vi "Set Transfer Line Valve Interlock Configuration.vi"(8 "error in (no error)":errorcluster, 9 "Manual Mode (False)":bool, 10 "Open? (False)":bool, 11 "Preparation Line in":refnum<class "Preparation Line.lvclass">) -> (0 "error out":errorcluster, 1 "Interlock Chain":refnum<class "Interlock Chain.lvclass">, 2 "Open? (False)":bool, 3 "Preparation Line out":refnum<class "Preparation Line.lvclass">)   [LabVIEW 2015, in "cRIO-Carbondioxide.lvlib" / "CO2-Actor.lvlib" / "Preparation Line.lvclass"]
uses:
  Preparation Line.lvclass
  Interlocks/Interlock Chain/Interlock Chain.lvclass
  Interlocks/Interlock/Interlock.lvclass
  Interlocks/Controls/Add IL to -Enumerator.ctl
  Transfer Line/Transfer Line.lvclass
  Interlocks/Interlock Sample/Interlock Sample.lvclass
  subs/Sample/Sample.lvclass
  CO2 Actor Messages/Ping Msg/Ping Msg.lvclass/Ping Msg.ctl
  <vilib>/ActorFramework/Message Enqueuer/Message Enqueuer.lvclass/Message Enqueuer.ctl
  Transfer Line/Transfer Line.lvclass/Transfer Line.ctl
  Interlocks/Interlock Chain/Interlock Chain.lvclass/Interlock Chain.ctl
  <vilib>/ActorFramework/Message Enqueuer/Enqueue.vi
  <vilib>/ActorFramework/Message Priority Queue/Priority Enqueue.vi
  subs/Sample/Read Sample From Container.vi
  CO2 Actor Messages/Ping Msg/Ping Msg.lvclass
  <vilib>/ActorFramework/Actor/Actor.lvclass
  CO2 Actor/CO2 Actor.lvclass
  cRIO-CO2/cRIO-CO2.lvclass
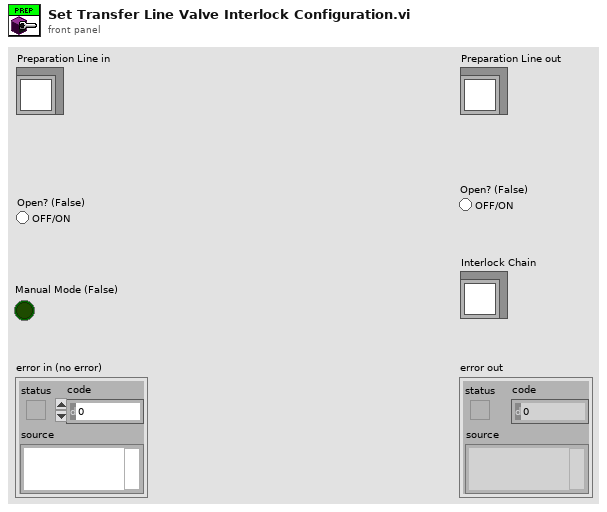
[diagram p1: front panel]
types:
  T1 = typedef "Add IL to -Enumerator.ctl" = enum16{"Deny", "Allow", "None"}
  T2 = typedef "Dedicated Enqueuers.ctl" = cluster{"Freezers":cluster{"Syringe":refnum<class "Message Enqueuer.lvclass">, "Tank 1":refnum<class "Message Enqueuer.lvclass">, "Tank 2":refnum<class "Message Enqueuer.lvclass">, "Tank 3":refnum<class "Message Enqueuer.lvclass">, "Tank 4":refnum<class "Message Enqueuer.lvclass">}, "Heaters":cluster{"Syringe":refnum<class "Message Enqueuer.lvclass">, "Piston":refnum<class "Message Enqueuer.lvclass">}, "Blowers":cluster{"Tank 1":refnum<class "Message Enqueuer.lvclass">, "Tank 2":refnum<class "Message Enqueuer.lvclass">, "Tank 3":refnum<class "Message Enqueuer.lvclass">, "Tank 4":refnum<class "Message Enqueuer.lvclass">, "Syringe":refnum<class "Message Enqueuer.lvclass">}, "Sample Line":refnum<class "Message Enqueuer.lvclass">, "Storage Line":refnum<class "Message Enqueuer.lvclass">, "Transfer Line":refnum<class "Message Enqueuer.lvclass">, "Syringe Stepper":refnum<class "Message Enqueuer.lvclass">, "Syringe Line":refnum<class "Message Enqueuer.lvclass">, "Capillary Line":refnum<class "Message Enqueuer.lvclass">, "Preparation Line":refnum<class "Message Enqueuer.lvclass">, "Turbo":refnum<class "Message Enqueuer.lvclass">, "Vacuum":refnum<class "Message Enqueuer.lvclass">, "He Line":refnum<class "Message Enqueuer.lvclass">, "Cylinder":refnum<class "Message Enqueuer.lvclass">}
  T3 = typedef "Sample Container.ctl" = cluster{"Sample In":refnum<k21>, "Sample Name":refnum<k21>, "Ti Cathode":refnum<k21>, "SampleQ":refnum<queue>}
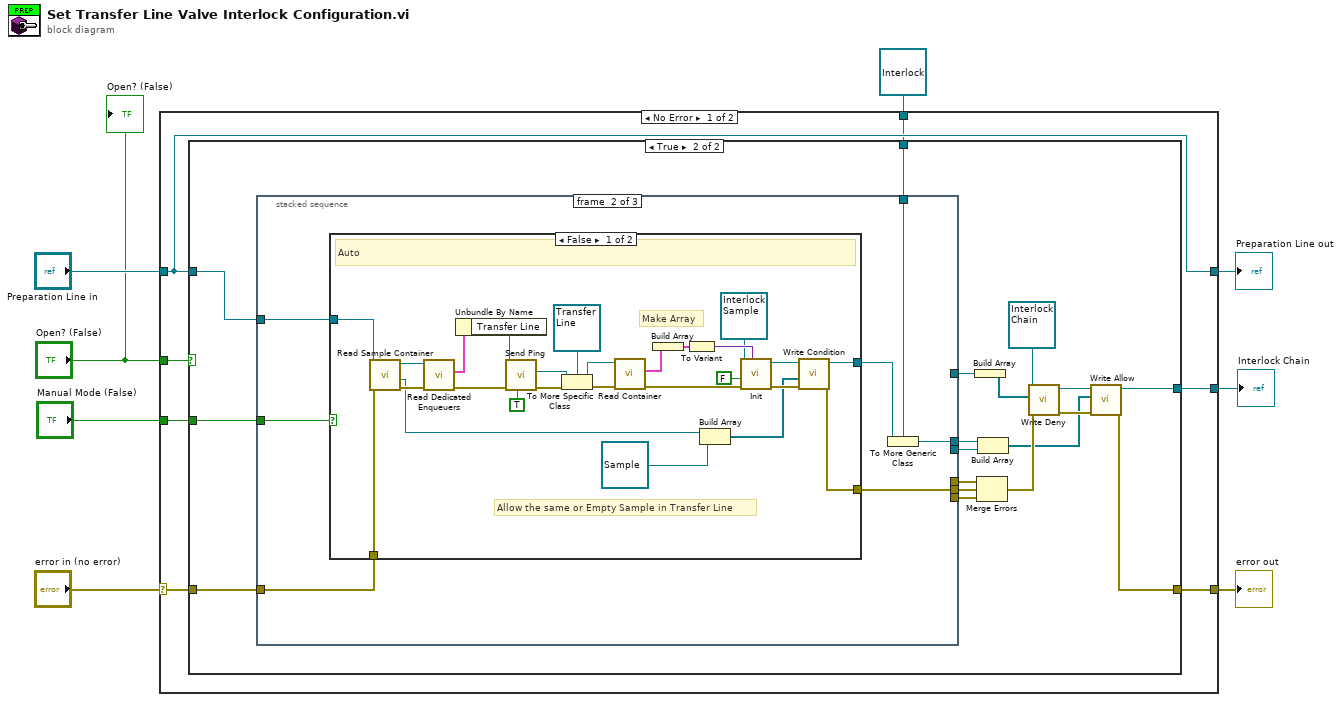
[diagram p0: block diagram]
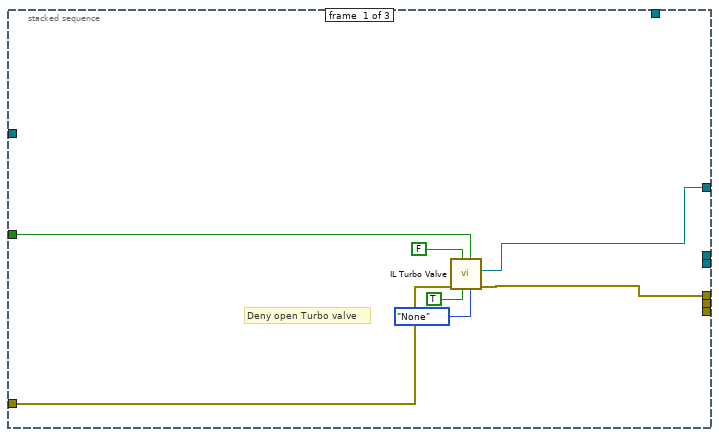
[diagram p3: hidden frame]
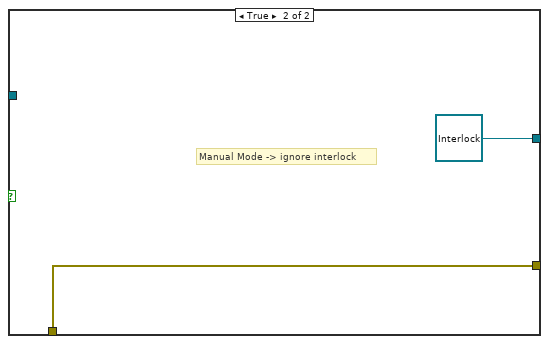
[diagram p4: hidden frame]
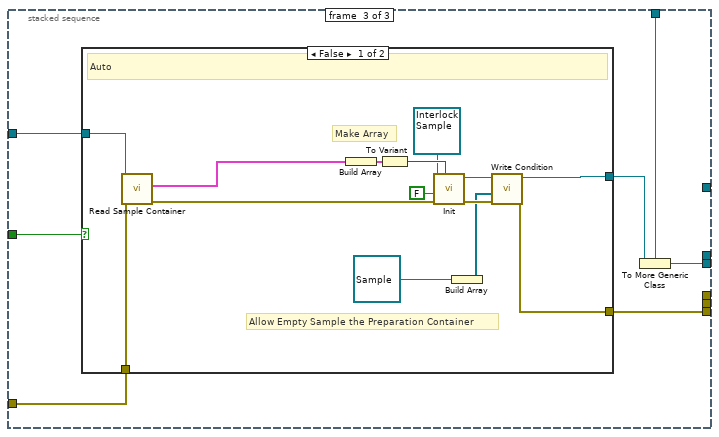
[diagram p5: hidden frame]
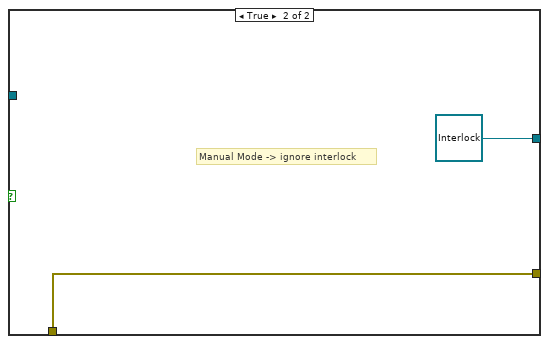
[diagram p6: hidden frame]
diagram:
  n1 = case shown="No Error" "error in (no error)" {
    selector: "error in (no error)" -> [w14 w101]
    tunnel: [w12 w101] -> w7
    tunnel: [w11 w100] -> w5
    tunnel: "Preparation Line in" -> [w11 w100]
    tunnel: "Manual Mode (False)" -> [w15 _]
    tunnel: [w13 _] -> w3
    tunnel: refnum<class "Interlock.lvclass"> refnum ("Interlock.lvclass") -> [w10 _]
    tunnel: "Open? (False)" -> [w9 _]
    frame No Error {
      n2 = case shown="True" w9 {
        tunnel: w15 -> [_ w34]
        tunnel: w14 -> [w16 w33]
        tunnel: [_ w30] -> w13
        tunnel: [w16 w29] -> w12
        tunnel: w11 -> [_ w23]
        tunnel: w10 -> [_ w22]
        frame False {
          # "Close Valve, no interlock"
        }
        frame True {
          n3 = stacked-sequence {
            tunnel: w34 -> [w37 w48 w83]
            tunnel: w23 -> [_ w47 w82]
            tunnel: w33 -> [w41 w46 w81]
            tunnel: [w39 _ _] -> w28
            tunnel: [w40 _ _] -> w26
            tunnel: w22 -> [_ w44 w79]
            tunnel: [_ w43 _] -> w20
            tunnel: [_ w42 _] -> w21
            tunnel: [_ _ w78] -> w18
            tunnel: [_ _ w77] -> w17
            frame #0 {
              # "Deny open Turbo valve"
              n4 = call "IL Turbo Valve.vi"("Add to (Deny)"=Add_IL_to_-Enumerator."None", "Ignore (F)"=w37, "Interlock Condition (ON/OFF)"=TRUE, "Stop Self on IL? (T)"=FALSE, "error in (no error)"=w41) -> ("error out"=w40:errorcluster, "IL Turbo Valve"=w39:refnum<class "Interlock.lvclass">)  [unwired: 4 in, 1 out]
            }
            frame #1 {
              n5 = case shown="False" w48 {
                tunnel: [w51 w76] -> w42
                tunnel: w47 -> [w69 _]
                tunnel: w46 -> [w67 w76]
                tunnel: [w50 refnum<class "Interlock.lvclass"> refnum ("Interlock.lvclass")] -> w45
                frame False {
                  # "Allow the same or Empty Sample in Transfer Line"
                  # "Make Array"
                  # "Auto"
                  n6 = call "Read Sample Container.vi"("error in (no error)"=w67, "Preparation Line in"=w69) -> ("error out"=w65:errorcluster, "Sample"=w53:refnum<class "Sample.lvclass">, "Preparation Line out"=w68:refnum<class "Preparation Line.lvclass">)  [unwired: 6 in, 1 out]
                  n7 = call "Read Dedicated Enqueuers.vi"("error in (no error)"=w65, "CO2 Actor in"=w68) -> ("error out"=w64:errorcluster, "Dedicated Enqueuers"=w74:T2)  [unwired: 6 in, 2 out]
                  n8 = Unbundle By Name(w74) -> ("Transfer Line"=w73:refnum<class "Message Enqueuer.lvclass">)
                  n9 = call "Send Ping.vi"("Return Self (F)"=TRUE, "error in (no error)"=w64, "Message Enqueuer"=w73) -> ("error out"=w71:errorcluster, "Actor out"=w70:refnum<class "Actor.lvclass">)  [unwired: 5 in, 2 out]
                  n10 = To More Specific Class(target class=refnum<class "Transfer Line.lvclass"> refnum ("Transfer Line.lvclass"), reference=w70, error in=w71) -> (specific class reference=w62:refnum<class "Transfer Line.lvclass">, error out=w63:errorcluster)
                  n11 = call "Read Container.vi"("error in (no error)"=w63, "Transfer Line in"=w62) -> ("error out"=w57:errorcluster, "Sample Container"=w60:T3)  [unwired: 5 in, 3 out]
                  n12 = Build Array(w60) -> (w61:T3[])
                  n13 = To Variant(anything=w61) -> (Variant=w56:variant)
                  n14 = Build Array(w53, refnum<class "Sample.lvclass"> refnum ("Sample.lvclass")) -> (w52:refnum<class "Sample.lvclass">[])
                  n15 = call-dynamic "Init.vi"("Sample Containers SHV (Array!)"=w56, "error in (no error)"=w57, "Stop Self on IL? (T)"=FALSE, "Interlock Sample in"=refnum<class "Interlock Sample.lvclass"> refnum ("Interlock Sample.lvclass")) -> ("error out"=w58:errorcluster, "Interlock Sample out"=w59:refnum<class "Interlock Sample.lvclass">)  [unwired: 6 in]
                  n16 = call "Write Condition.vi"("error in (no error)"=w58, "Samples"=w52, "Interlock Sample in"=w59) -> ("error out"=w51:errorcluster, "Interlock Sample out"=w50:refnum<class "Interlock Sample.lvclass">)  [unwired: 7 in]
                }
                frame True {
                  # "Manual Mode -> ignore interlock"
                }
              }
              n17 = To More Generic Class(target class=w44, reference=w45) -> (generic class reference=w43:refnum<class "Interlock.lvclass">)
            }
            frame #2 {
              n18 = case shown="False" w83 {
                tunnel: [w88 w99] -> w77
                tunnel: w82 -> [w97 _]
                tunnel: w81 -> [w96 w99]
                tunnel: [w87 refnum<class "Interlock.lvclass"> refnum ("Interlock.lvclass")] -> w80
                frame False {
                  # "Allow Empty Sample the Preparation Container"
                  # "Make Array"
                  # "Auto"
                  n19 = call "Read Sample Container.vi"("error in (no error)"=w96, "Preparation Line in"=w97) -> ("error out"=w86:errorcluster, "Container"=w85:T3)  [unwired: 6 in, 2 out]
                  n20 = Build Array(w85) -> (w95:T3[])
                  n21 = To Variant(anything=w95) -> (Variant=w92:variant)
                  n22 = call-dynamic "Init.vi"("Sample Containers SHV (Array!)"=w92, "error in (no error)"=w86, "Stop Self on IL? (T)"=FALSE, "Interlock Sample in"=refnum<class "Interlock Sample.lvclass"> refnum ("Interlock Sample.lvclass")) -> ("error out"=w93:errorcluster, "Interlock Sample out"=w94:refnum<class "Interlock Sample.lvclass">)  [unwired: 6 in]
                  n23 = Build Array(refnum<class "Sample.lvclass"> refnum ("Sample.lvclass")) -> (w89:refnum<class "Sample.lvclass">[])
                  n24 = call "Write Condition.vi"("error in (no error)"=w93, "Samples"=w89, "Interlock Sample in"=w94) -> ("error out"=w88:errorcluster, "Interlock Sample out"=w87:refnum<class "Interlock Sample.lvclass">)  [unwired: 7 in]
                }
                frame True {
                  # "Manual Mode -> ignore interlock"
                }
              }
              n25 = To More Generic Class(target class=w79, reference=w80) -> (generic class reference=w78:refnum<class "Interlock.lvclass">)
            }
          }
          n26 = Build Array(w28) -> (w27:refnum<class "Interlock.lvclass">[])
          n27 = Merge Errors(w26, w21, w17) -> (w25:errorcluster)
          n28 = Build Array(w20, w18) -> (w19:refnum<class "Interlock.lvclass">[])
          n29 = call "Write Deny.vi"("error in (no error)"=w25, "Deny"=w27, "Interlock Chain in"=refnum<class "Interlock Chain.lvclass"> refnum) -> ("error out"=w24:errorcluster, "Interlock Chain out"=w32:refnum<class "Interlock Chain.lvclass">)  [unwired: 7 in]
          n30 = call "Write Allow.vi"("error in (no error)"=w24, "Allow"=w19, "Interlock Chain in"=w32) -> ("error out"=w29:errorcluster, "Interlock Chain out"=w30:refnum<class "Interlock Chain.lvclass">)  [unwired: 7 in]
        }
      }
    }
    frame Error {
    }
  }
  "error out" <- w7
  "Preparation Line out" <- w5
  "Interlock Chain" <- w3
  "Open? (False)" <- "Open? (False)"
